vi "Create Message Queues.vi"(8 "error in (no error)":errorcluster) -> (0 "error out":errorcluster, 3 "Message Queues out":T1)   [LabVIEW 2016, in "Trace Grabber.lvlib"]
uses:
  Trace Grabber/Trace Grabber.lvlib
  Message Queues.ctl
  Message.ctl
  Enqueue Message (Single).vi
  Message Queue.lvlib
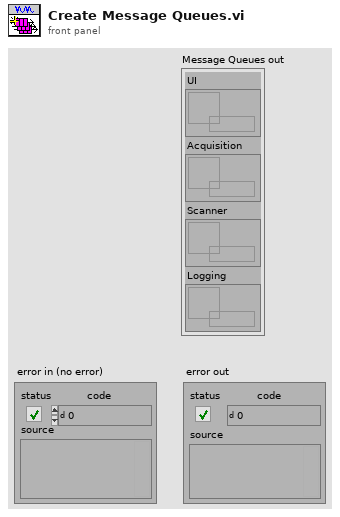
[diagram p1: front panel]
types:
  T1 = typedef "Trace Grabber.lvlib/Message Queues.ctl" = cluster{"UI":refnum<queue>, "Acquisition":refnum<queue>, "Scanner":refnum<queue>, "Logging":refnum<queue>}
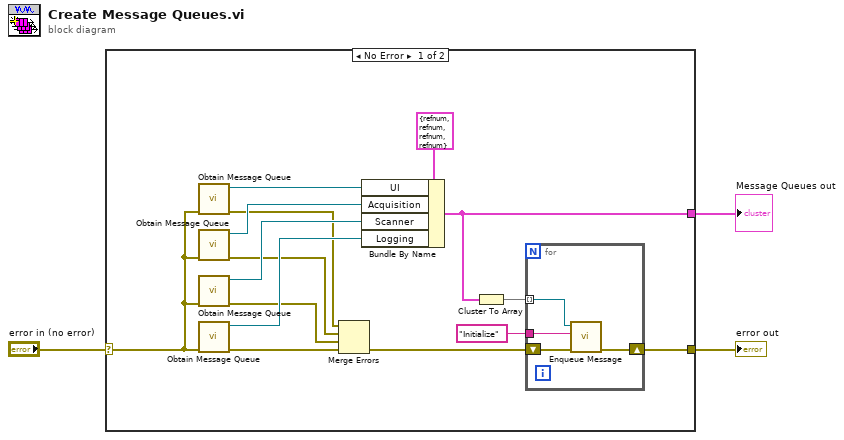
[diagram p0: block diagram]
diagram:
  n1 = case shown="No Error" "error in (no error)" {
    selector: "error in (no error)" -> [w13 w23]
    tunnel: [w5 w23] -> w2
    tunnel: [w8 _] -> w1
    frame No Error {
      n2 = call "Obtain Message Queue.vi"("error in (no error)"=w13) -> ("error out"=w11:errorcluster, "Message Queue out"=w18:refnum<queue>)  [unwired: 9 in]
      n3 = call "Obtain Message Queue.vi"("error in (no error)"=w13) -> ("error out"=w10:errorcluster, "Message Queue out"=w16:refnum<queue>)  [unwired: 9 in]
      n4 = call "Obtain Message Queue.vi"("error in (no error)"=w13) -> ("error out"=w9:errorcluster, "Message Queue out"=w15:refnum<queue>)  [unwired: 9 in]
      n5 = call "Obtain Message Queue.vi"("error in (no error)"=w13) -> ("error out"=w12:errorcluster, "Message Queue out"=w14:refnum<queue>)  [unwired: 9 in]
      n6 = Merge Errors(w11, w10, w9, w12) -> (w6:errorcluster)
      n7 = Bundle By Name(cluster=T1 {"UI"=refnum, "Acquisition"=refnum, "Scanner"=refnum, "Logging"=refnum} ("input cluster"), "UI"=w18, "Acquisition"=w16, "Scanner"=w15, "Logging"=w14) -> (w8:T1)
      n8 = Cluster To Array(cluster=w8) -> (array=w7:refnum<queue>[])
      n9 = for {
        tunnel: w7 -> [w22] mode=indexing
        shift-right: [w20] -> w5
        shift-left: w6 -> [w21]
        tunnel: "Initialize" ("State") -> [w19]
        n10 = call-poly "Enqueue Message.vi"("error in (no error)"=w21, "State"=w19, "Message Queue in"=w22) -> ("error out"=w20:errorcluster)  [unwired: 7 in, 1 out]
      }
    }
    frame Error {
    }
  }
  "error out" <- w2
  "Message Queues out" <- w1
